vi "Set acquiring.vi"(8 "error in (no error)":errorcluster, 10 "is acquiring?":bool, 11 "DAQMH121119OrcaFlash in":refnum<class "DAQOrcaFlash.lvclass">) -> (0 "error out":errorcluster, 3 "DAQMH121119OrcaFlash out":refnum<class "DAQOrcaFlash.lvclass">)   [LabVIEW 2012, in "DAQOrcaFlash.lvclass"]
uses:
  DAQOrcaFlash.lvclass
  DAQOrcaFlash.lvclass/DAQOrcaFlash.ctl
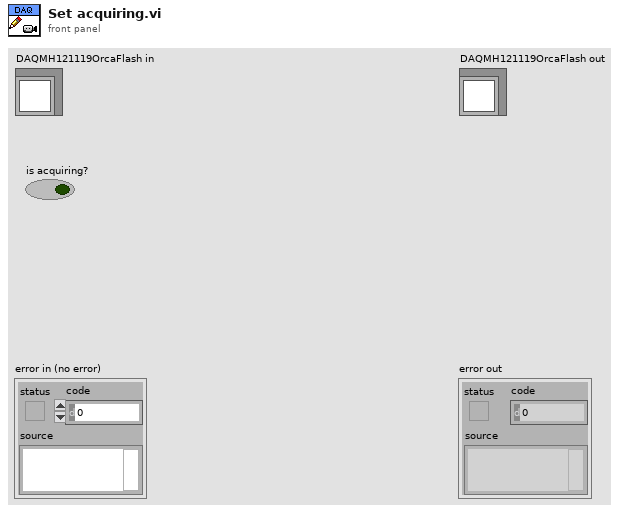
[diagram p1: front panel]
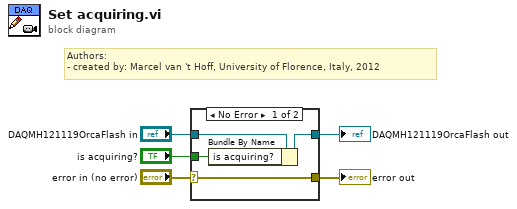
[diagram p0: block diagram]
diagram:
  # "Authors: \n- created by: Marcel van 't Hoff, University of Florence, Italy, 2012"
  n1 = case shown="No Error" "error in (no error)" {
    selector: "error in (no error)" -> [w9 w11]
    tunnel: [w9 w11] -> w4
    tunnel: [w7 w10] -> w2
    tunnel: "DAQMH121119OrcaFlash in" -> [w8 w10]
    tunnel: "is acquiring?" -> [w6 _]
    frame No Error {
      n2 = Bundle By Name(cluster=w8, "is acquiring?"=w6) -> (w7:refnum<class "DAQOrcaFlash.lvclass">)
    }
    frame Error {
    }
  }
  "error out" <- w4
  "DAQMH121119OrcaFlash out" <- w2
